vi "getIndex_temp.vi"(8 "error in (no error)":errorcluster, 9 "value":string, 10 "key":string, 11 "VElement":variant) -> (0 "error out":errorcluster, 3 "indexOut":i32)   [LabVIEW 2015]
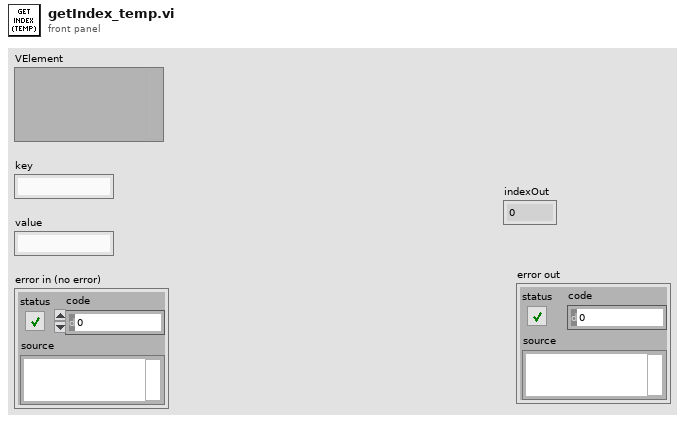
[diagram p1: front panel]
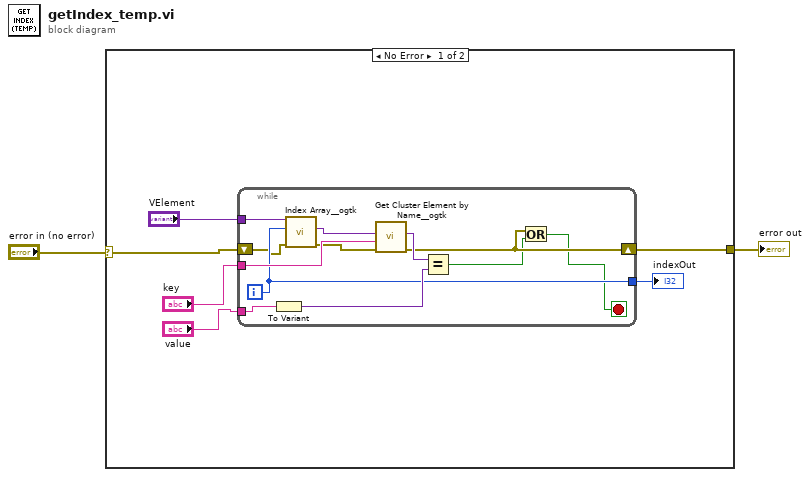
[diagram p0: block diagram]
diagram:
  n1 = case shown="No Error" "error in (no error)" {
    selector: "error in (no error)" -> [w7 w21]
    tunnel: [w3 w21] -> w1
    frame No Error {
      n2 = while {
        tunnel: "VElement" -> [w20]
        tunnel: "key" -> [w18]
        tunnel: "value" -> [w17]
        tunnel: [w14] -> w6
        shift-right: [w13] -> w3
        shift-left: w7 -> [w10]
        i -> [w14]
        stop <- w11 stop-if-true
        n3 = To Variant(anything=w17) -> (Variant=w15:variant)
        n4 = call <userlib>:"Index Array__ogtk.vi"("error in (no error)"=w10, "Index (1D)"=w14, "MultiD Array"=w20) -> ("error out"=w9:errorcluster, "Array Element"=w19:variant)  [unwired: 7 in]
        n5 = call <userlib>:"Get Cluster Element by Name__ogtk.vi"("error in (no error)"=w9, "Element Name"=w18, "Cluster"=w19) -> ("error out"=w13:errorcluster, "VElement"=w16:variant)  [unwired: 6 in, 1 out]
        n6 = Equal?(x=w16, y=w15) -> (x = y?=w12:bool)
        n7 = Or(x=w13, y=w12) -> (x .or. y?=w11:bool)
      }
      "indexOut" <- w6
    }
    frame Error {
    }
  }
  "error out" <- w1
